vi "motor_initialize.vi"(4 "error in (no error)":errorcluster, 6 "Request data":variant, 7 "Python session in":refnum<k35>) -> (0 "error out":errorcluster, 2 "Response data":variant, 3 "Python session out":refnum<k35>)   [LabVIEW 2022 SP3]
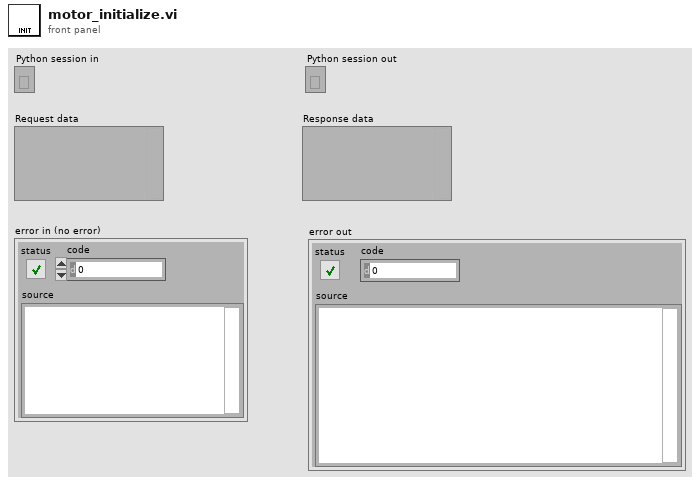
[diagram p1: front panel]
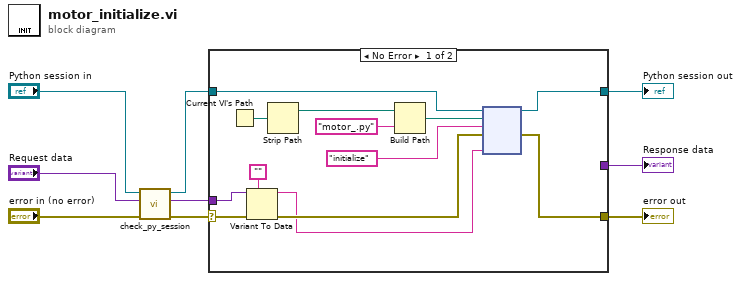
[diagram p0: block diagram]
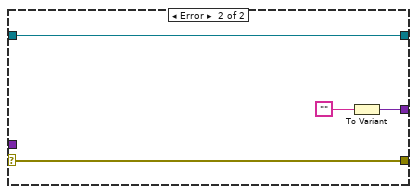
[diagram p2: hidden frame]
diagram:
  n1 = call "check_py_session.vi"("error in"="error in (no error)", "Request data"="Request data", "Python session in"="Python session in") -> ("error out"=w3:errorcluster, "Response data"=w4:variant, "Python session out"=w5:refnum<k35>)  [unwired: 2 in]
  n2 = case shown="No Error" w3 {
    selector: w3 -> [w13 w26]
    tunnel: w5 -> [w22 w25]
    tunnel: [w16 w25] -> w9
    tunnel: w4 -> [w14 _]
    tunnel: [w11 w26] -> w2
    tunnel: [_ w23] -> w1
    frame No Error {
      n3 = Current VI's Path() -> (path=w18:path)
      n4 = Variant To Data(error in=w13, type="", Variant=w14) -> (data=w10:string, error out=w12:errorcluster)
      n5 = Strip Path(path=w18) -> (stripped path=w17:path)  [unwired: 1 out]
      n6 = Build Path(base path=w17, name or relative path="motor_.py") -> (appended path=w20:path)
      n7 = node(w22, w20, "initialize" ("function name"), w12, w10) -> (w16:refnum<k35>, w11:errorcluster)  [unwired: 3 in, 2 out]
    }
    frame Error {
      n8 = To Variant(anything="") -> (Variant=w23:variant)
    }
  }
  "error out" <- w2
  "Python session out" <- w9
  "Response data" <- w1
